vi "PV Diaphragm Pumps Control commands .vi"(8 "error in (no error)":errorcluster, 9 "MVP Control commands - Cluster":T1={"Parameter"=enum."Standby [002]", "Parameter\nread only<->describe"=FALSE, "off        on"=TRUE, "Purge mode"=0, "Control via interface"=2, "Configuration DO2 / DO1"=0} caption="Operating adjustment - Cluster" {"Control via interface" items=["remote"=1, "RS 485"=2, "PV.can"=4, "Unlock the interface selection"=255]; "Configuration DO2 / DO1" items=["1 = no error"=1, "2 = error"=2, "5 = target speed is reached"=5, "6 = pump on"=6, "9 = \"0\""=9, "10 = \"1\""=10, "11 = remote priority active"=11]; "Purge mode" items=["auto", "closed", "open"]}, 10 "Adress of unit":u16=1 min=1 max=999 step=1, 11 "VISA session":refnum<visa-resource-name>) -> (0 "error out":errorcluster, 2 "response (data)":string, 3 "dup VISA session":refnum<visa-resource-name>)   [LabVIEW 2021, in "Pfeiffer Vacuum.lvlib"]
doc: "There are 10 parameters available, only one of which can be enabled at a time. \n\nStandby [002]\nFault acknowledgment [009]\nPump [010]\nCongiguration output DO2 [019]\nCongiguration output DO1 [024]\nSeed setting mode [026]\nPurge gas configuration [030]\nPurge gas [050]\nControl via interface [060]\nInterface selection locked [061]\n\n\nNote: The controls right of this one will set the appropriate values for the selected parameter. Any settings for an parameter that is not selected will be ignored. If a value is out of range, it will be changed to either the upper or the lower limit of the range."
uses:
  <instrlib>/Pfeiffer Vacuum/Pfeiffer Vacuum.lvlib
  <instrlib>/Pfeiffer Vacuum/Public/DiaphragmPumps/PV Diapdragm Pumps Control commands - Cluster.ctl
panel:
  # "Standby                                   \n Pump \n Speed setting mode \n Purge gas\n Interface selection locked"
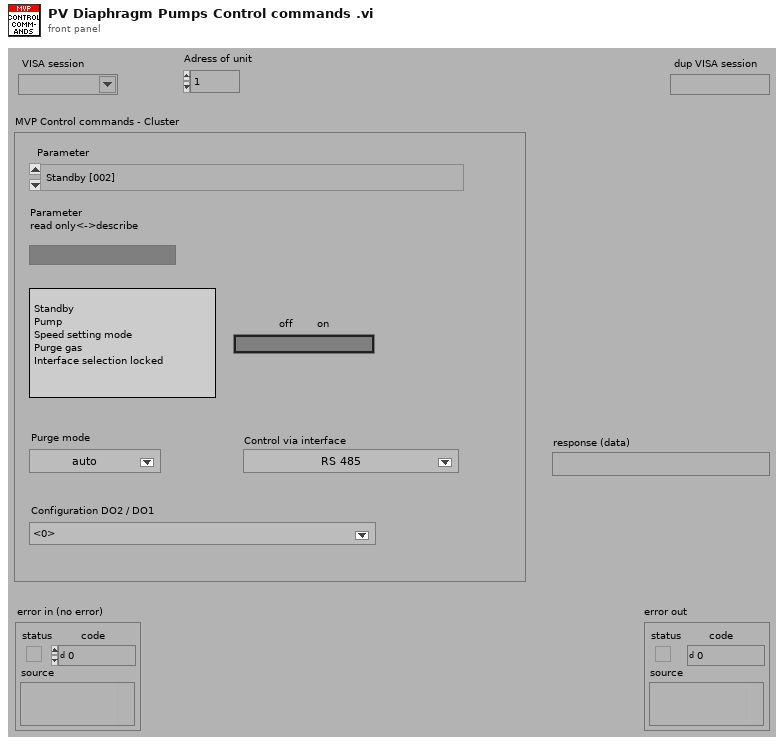
[diagram p1: front panel]
types:
  T1 = typedef "Pfeiffer Vacuum.lvlib/PV Diapdragm Pumps Control commands - Cluster.ctl" = cluster{"Parameter":enum16{"Standby [002]", "Fault acknowledgment [009]", "Pump [010]", "Configuration output DO2 [019]", "Configuration output DO1 [024]", "Speed setting mode [026]", "Purge gas configuration [030]", "Purge gas [050]", "Control via interface [060]", "Interface selection locked [061]"}, "Parameter\nread only<->describe":bool, "off        on":bool, "Purge mode":u16, "Control via interface":u16, "Configuration DO2 / DO1":u16}
  T2 = enum16{"Standby [002]", "Fault acknowledgment [009]", "Pump [010]", "Configuration output DO2 [019]", "Configuration output DO1 [024]", "Speed setting mode [026]", "Purge gas configuration [030]", "Purge gas [050]", "Control via interface [060]", "Interface selection locked [061]"}
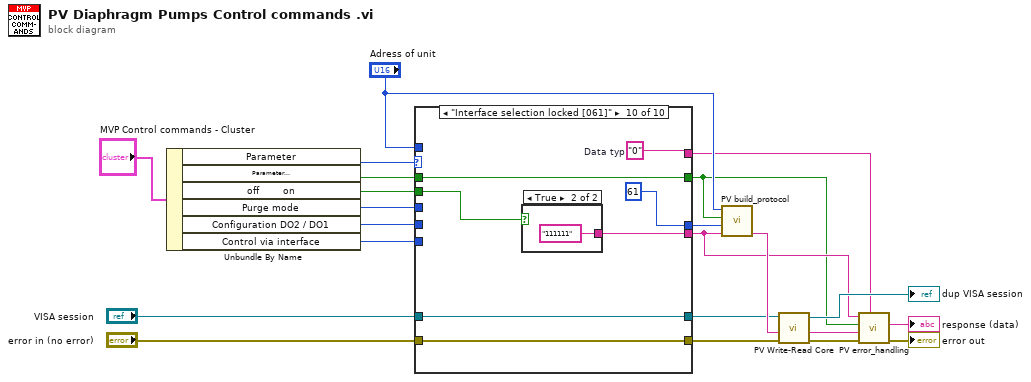
[diagram p0: block diagram]
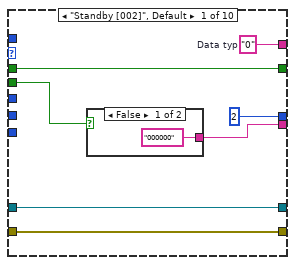
[diagram p2: hidden frame]
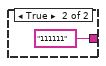
[diagram p3: hidden frame]
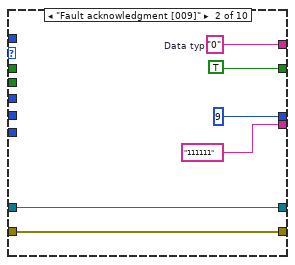
[diagram p4: hidden frame]
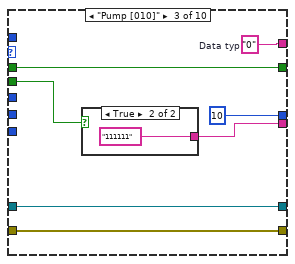
[diagram p5: hidden frame]
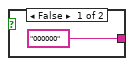
[diagram p6: hidden frame]
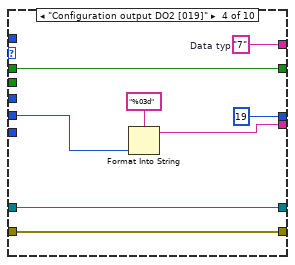
[diagram p7: hidden frame]
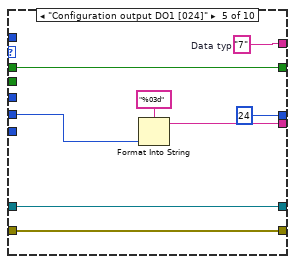
[diagram p8: hidden frame]
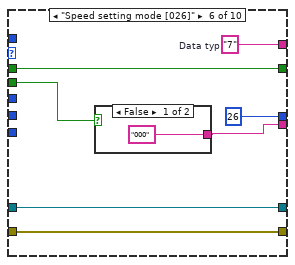
[diagram p9: hidden frame]
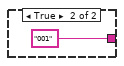
[diagram p10: hidden frame]
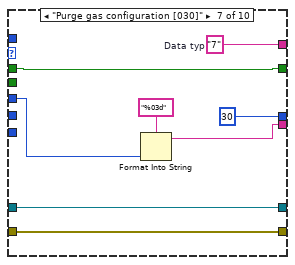
[diagram p11: hidden frame]
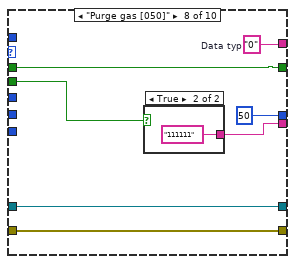
[diagram p12: hidden frame]
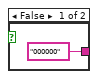
[diagram p13: hidden frame]
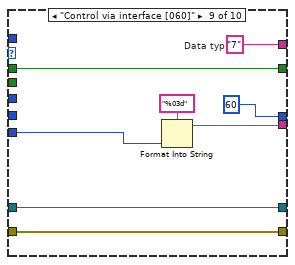
[diagram p14: hidden frame]
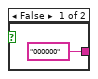
[diagram p15: hidden frame]
diagram:
  n1 = Unbundle By Name("MVP Control commands - Cluster") -> ("Parameter"=w21:T2, "Parameter\nread only<->describe"=w20:bool, "off        on"=w4:bool, "Purge mode"=w2:u16, "Configuration DO2 / DO1"=w3:u16, "Control via interface"=w1:u16)
  n2 = case shown="\"Interface selection locked [061]\"" w21 {
    tunnel: [u16 2 ("Parameter-number") u16 9 ("Parameter-number") u16 10 ("Parameter-number") u16 19 ("Parameter-number") u16 24 ("Parameter-number") u16 26 ("Parameter-number") u16 30 ("Parameter-number") u16 50 ("Parameter-number") u16 60 ("Parameter-number") u16 61 ("Parameter-number")] -> w22
    tunnel: [w28 "111111" ("Data") w43 w48 w56 w64 w72 w80 w90 w99] -> w10
    tunnel: [w27 TRUE w42 w54 w61 w65 w76 w83 w92 w98] -> w8
    tunnel: w20 -> [w27 _ w42 w54 w61 w65 w76 w83 w92 w98]
    tunnel: w4 -> [w26 _ w41 _ _ w63 _ w81 _ w97]
    tunnel: [w25 w35 w40 w53 w60 w67 w75 w84 w93 w101] -> w9
    tunnel: "VISA session" -> [w24 w34 w39 w52 w59 w69 w79 w86 w96 w103]
    tunnel: [w24 w34 w39 w52 w59 w69 w79 w86 w96 w103] -> w15
    tunnel: "Adress of unit" -> [_ _ _ _ _ _ _ _ _ _]
    tunnel: "error in (no error)" -> [w23 w33 w38 w51 w58 w68 w78 w85 w95 w102]
    tunnel: [w23 w33 w38 w51 w58 w68 w78 w85 w95 w102] -> w14
    tunnel: w3 -> [_ _ _ w47 w55 _ _ _ _ _]
    tunnel: w2 -> [_ _ _ _ _ _ w73 _ _ _]
    tunnel: w1 -> [_ _ _ _ _ _ _ _ w89 _]
    frame "Standby [002]", Default {
      w25 = "0"  # Data typ
      n3 = case shown="False" w26 {
        tunnel: ["000000" ("Data") "111111" ("Data")] -> w28
        frame False {
        }
        frame True {
        }
      }
    }
    frame "Fault acknowledgment [009]" {
      w35 = "0"  # Data typ
    }
    frame "Pump [010]" {
      w40 = "0"  # Data typ
      n4 = case shown="True" w41 {
        tunnel: ["000000" ("Data") "111111" ("Data")] -> w43
        frame False {
        }
        frame True {
        }
      }
    }
    frame "Configuration output DO2 [019]" {
      w53 = "7"  # Data typ
      n5 = Format Into String(format string="%03d" ("Format-String"), w47) -> (resulting string=w48:string)  [unwired: 2 in, 1 out]
    }
    frame "Configuration output DO1 [024]" {
      w60 = "7"  # Data typ
      n6 = Format Into String(format string="%03d" ("Format-String"), w55) -> (resulting string=w56:string)  [unwired: 2 in, 1 out]
    }
    frame "Speed setting mode [026]" {
      w67 = "7"  # Data typ
      n7 = case shown="False" w63 {
        tunnel: ["000" ("Data") "001" ("Data")] -> w64
        frame False {
        }
        frame True {
        }
      }
    }
    frame "Purge gas configuration [030]" {
      w75 = "7"  # Data typ
      n8 = Format Into String(format string="%03d" ("Format-String"), w73) -> (resulting string=w72:string)  [unwired: 2 in, 1 out]
    }
    frame "Purge gas [050]" {
      w84 = "0"  # Data typ
      n9 = case shown="True" w81 {
        tunnel: ["000000" ("Data") "111111" ("Data")] -> w80
        frame False {
        }
        frame True {
        }
      }
    }
    frame "Control via interface [060]" {
      w93 = "7"  # Data typ
      n10 = Format Into String(format string="%03d" ("Format-String"), w89) -> (resulting string=w90:string)  [unwired: 2 in, 1 out]
    }
    frame "Interface selection locked [061]" {
      w101 = "0"  # Data typ
      n11 = case shown="True" w97 {
        tunnel: ["000000" ("Data") "111111" ("Data")] -> w99
        frame False {
        }
        frame True {
        }
      }
    }
  }
  n12 = call <instrlib>:"PV build_protocol.vi"("Data"=w10, "Parameter-number"=w22, "parameter\nread<->describe"=w8, "Adress"="Adress of unit") -> ("output"=w16:string)  [unwired: 3 in]
  n13 = call <instrlib>:"PV Write-Read Core.vi"("error in"=w14, "Write data in"=w16, "VISA session"=w15) -> ("error out"=w12:errorcluster, "response (data) out"=w13:string, "dup VISA session"=→"dup VISA session":refnum<visa-resource-name>)  [unwired: 2 in]
  n14 = call <instrlib>:"PV error_handling.vi"("Data Typ in"=w9, "error in"=w12, "response (data) in"=w13, "Parameter\nread only<->describe"=w8, "data in"=w10) -> ("error out"=→"error out":errorcluster, "Data out"=→"response (data)":string)  [unwired: 4 in, 1 out]
